vi "Fluke 525B.vi"(1 "Primary Value (1.234)":dbl format="%^.3e", 2 "error in (no error)":errorcluster, 3 "Output Value(s) (3: Volts ac or volts dc with 0 Hz)":u32(ring)=11 items=["Amplitude", "Volts dc or update volts ac", "Volts ac dBm update", "Volts ac or volts dc with 0 Hz", "Volts ac in dBm", "Current dc or update current ac", "Current ac", "Update frequency", "Resistance", "Capacitance", "Temperature (Celsius)", "Temperature (Fahrenheit)", "Power dc or update power ac", "Power ac", "Dual volts dc or update dual ac", "Dual volts ac in volts", "Power ac in dBm update", "Power ac in dBm", "Dual volts ac in dBm update", "Dual volts ac in dBm"], 4 "VISA resource name":refnum<visa-resource-name>) -> (0 "error out":errorcluster)   [LabVIEW 2016]
doc: "This VI is a simple example on how to use the instrument driver. Following VIs are called:\n\n(1) Set Output Values (setOutputValues):\nThis VI sets the output of the Calibrator and establishes a new reference point for the error mode.\n\n(2) Wait-to-Continue (waitToContinue):\nThis VI Prevents further remote commands from being executed until all previous remote commands have been executed.\n\n(3) Set Output Mode (setOutputMode):\nThis VI activates or deactivates the Calibrator output if it is in standby or operate mode.\n\nRange checking, instrument model checking and option checking is performed by each of used VIs internaly. To skip instrument model checking, option checking and error checking, call VI\n\n State Checking.vi\n\nand disable it. When state checking is disabled driver does not check for correct instrument model or option to be used with each of VIs. This might cause unexpected behaviour of the instrument. Simpliest way how to disable state checking from the begining is calling initialization VI with the parameter ID Query = False. But this is not recommended as functionality of the driver depends on the instrument models and its options.\n\nNote:\n\nRefer also to the descriptions of used VIs."
uses:
  Fluke 5XXX Series Multicalibrators.lvlib
panel:
  in  "Output Mode (1: Operate)":u32(ring)=1 items=["Standby", "Operate"]
  in  "Fundamental Frequency (50.0 Hz)":dbl=50.0 format="%^.3e"
  in  "Secondary Value (0.0)":dbl format="%^.3e"
  # "(c) 2005-2012 National Instruments.  ALL RIGHTS RESERVED."
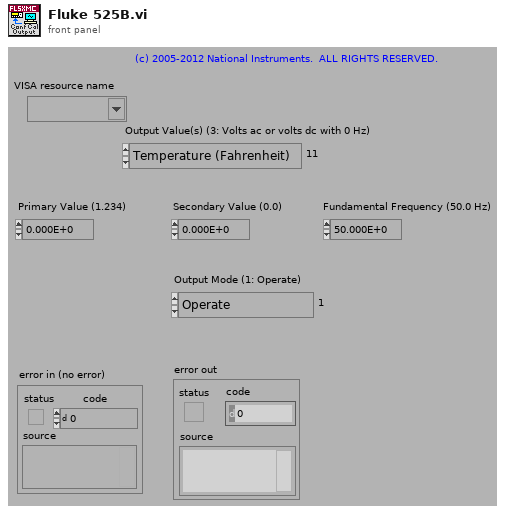
[diagram p1: front panel]
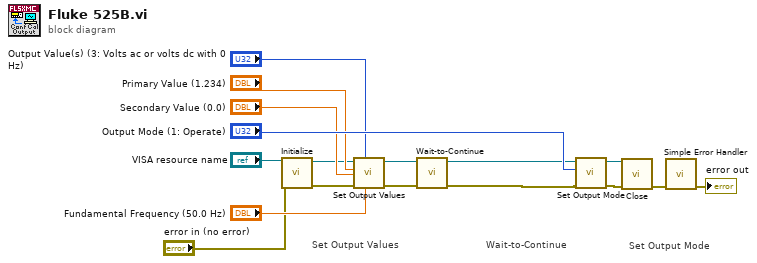
[diagram p0: block diagram]
diagram:
  # "Set Output Mode"
  # "Wait-to-Continue"
  # "Set Output Values"
  n1 = call "Initialize.vi"("VISA resource name"="VISA resource name", "error in (no error)"="error in (no error)") -> ("VISA resource name out"=w8:refnum<visa-resource-name>, "error out"=w9:errorcluster)  [unwired: 12 in]
  n2 = call "Set Output Values.vi"("Fundamental Frequency (0.0 Hz)"="Fundamental Frequency (50.0 Hz)", "Output Value(s) (0 - Amplitude)"="Output Value(s) (3: Volts ac or volts dc with 0 Hz)", "error in (no error)"=w9, "Secondary Value (0.0)"="Secondary Value (0.0)", "Primary Value (0.0)"="Primary Value (1.234)", "VISA resource name"=w8) -> ("error out"=w17:errorcluster, "VISA resource name out"=w16:refnum<visa-resource-name>)  [unwired: 4 in]
  n3 = call "Wait-to-Continue.vi"("error in (no error)"=w17, "VISA resource name"=w16) -> ("error out"=w3:errorcluster, "VISA resource name out"=w4:refnum<visa-resource-name>)  [unwired: 8 in]
  n4 = call "Set Output Mode.vi"("error in (no error)"=w3, "Output Mode (0: Standby)"="Output Mode (1: Operate)", "VISA resource name"=w4) -> ("error out"=w6:errorcluster, "VISA resource name out"=w7:refnum<visa-resource-name>)  [unwired: 7 in]
  n5 = call "Close.vi"("VISA resource name"=w7, "error in (no error)"=w6) -> ("error out"=w5:errorcluster)  [unwired: 13 in]
  n6 = call <vilib>:"Simple Error Handler.vi"("error in (no error)"=w5) -> ("error out"=→"error out":errorcluster)  [unwired: 4 in, 4 out]
